vi "Rio_Trapazodial_Velocity_Time.vi"(9 "Controls":T1={"Start Pos"=0.0, "End Pos"=0.0, "Max V R/m"=100, "Accel Time (S)"=0.0}, 11 "Error In":errorcluster) -> (0 "Forward (t)/Reverse (f)":bool, 1 "Waveform Graph":dbl[](graph), 3 "Error Out":errorcluster)   [LabVIEW 2017]
uses:
  <vilib>/Analysis/1siggen.llb/Ramp Pattern by Samples.vi
  <vilib>/Analysis/NI_AALBase.lvlib
panel:
  out "recalc Max v":dbl
  out "Accel R/S2":dbl
  out "d @ Max v":dbl
  out "Max V R/S":dbl
  out "Accel Samples":dbl
  out "No. Samples":dbl
  out "Time":dbl
  out "d Revs":dbl
  out "d Counts":i64
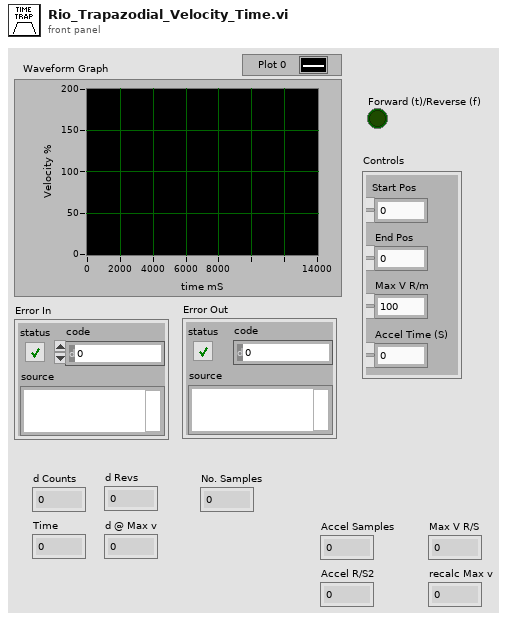
[diagram p1: front panel]
types:
  T1 = cluster{"Start Pos":dbl, "End Pos":dbl, "Max V R/m":i32, "Accel Time (S)":dbl}
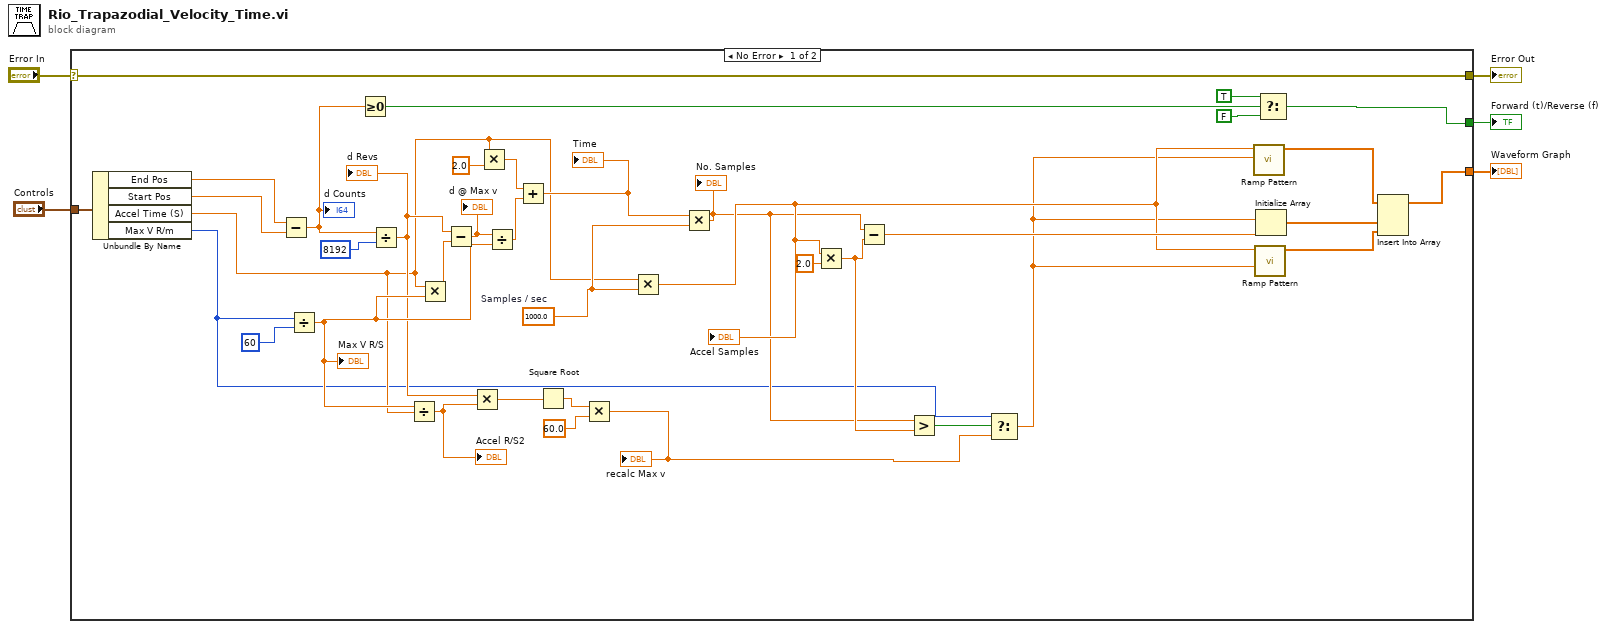
[diagram p0: block diagram]
diagram:
  n1 = case shown="No Error" "Error In" {
    selector: "Error In" -> [w41 w44]
    tunnel: [w43 _] -> w5
    tunnel: [w42 _] -> w4
    tunnel: [w41 w44] -> w2
    tunnel: "Controls" -> [w10 _]
    frame No Error {
      w26 = 1000.0  # Samples / sec
      n2 = Unbundle By Name(w10) -> ("End Pos"=w9:dbl, "Start Pos"=w8:dbl, "Accel Time (S)"=w7:dbl, "Max V R/m"=w6:i32)
      n3 = Subtract(x=w9, y=w8) -> (x-y=w33:dbl)
      "d Counts" <- w33
      n4 = Divide(x=w6, y=60) -> (x/y=w21:dbl)
      "Max V R/S" <- w21
      n5 = Greater Or Equal To 0?(x=w33) -> (x >= 0?=w32:bool)
      n6 = Divide(x=w33, y=i64 8192) -> (x/y=w19:dbl)
      "d Revs" <- w19
      n7 = Divide(x=w21, y=w7) -> (x/y=w20:dbl)
      "Accel R/S2" <- w20
      n8 = Multiply(x=w7, y=w21) -> (x*y=w25:dbl)
      n9 = Subtract(x=w19, y=w25) -> (x-y=w24:dbl)
      "d @ Max v" <- w24
      n10 = Multiply(x=w19, y=w20) -> (x*y=w18:dbl)
      n11 = Multiply(x=w7, y=2.0) -> (x*y=w29:dbl)
      n12 = Divide(x=w24, y=w21) -> (x/y=w28:dbl)
      n13 = Add(x=w29, y=w28) -> (x+y=w27:dbl)
      "Time" <- w27
      n14 = Square Root(x=w18) -> (sqrt(x)=w17:dbl)
      n15 = Multiply(x=w17, y=60.0) -> (x*y=w14:dbl)
      "recalc Max v" <- w14
      n16 = Multiply(x=w7, y=w26) -> (x*y=w22:dbl)
      "Accel Samples" <- w22
      n17 = Multiply(x=w27, y=w26) -> (x*y=w11:dbl)
      "No. Samples" <- w11
      n18 = Multiply(x=w22, y=2.0) -> (x*y=w12:dbl)
      n19 = Subtract(x=w11, y=w12) -> (x-y=w23:dbl)
      n20 = Greater?(x=w11, y=w12) -> (0:w13:bool)
      n21 = Select(t=w6, s=w13, f=w14) -> (s? t:f=w15:dbl)
      n22 = call-poly <vilib>:"Ramp Pattern.vi"("end"=w15, "samples"=w22) -> ("Ramp Pattern"=w38:dbl[])  [unwired: 8 in, 1 out]
      n23 = call-poly <vilib>:"Ramp Pattern.vi"("start"=w15, "samples"=w22) -> ("Ramp Pattern"=w37:dbl[])  [unwired: 8 in, 1 out]
      n24 = Initialize Array(w15, w23) -> (w34:dbl[])
      n25 = Select(t=TRUE, s=w32, f=FALSE) -> (s? t:f=w42:bool)
      n26 = Insert Into Array(array=w38, new element #1=w34, new element #2=w37) -> (w43:dbl[])  [unwired: 1 in]
    }
    frame Error {
    }
  }
  "Waveform Graph" <- w5
  "Forward (t)/Reverse (f)" <- w4
  "Error Out" <- w2
